vi "BasicHostExampleWithIFw.vi"() -> ()   [LabVIEW 2015]
uses:
  QuadEncInterface/Configuration.ctl
  <vilib>/FPGAPlugInAG/sbRIO-9607/niLvFpga_Open_sbRIO-9607.vi
  <vilib>/rvi/interface/common/dynamic/niFpgaDynamicAddResources.vi
  <vilib>/Utility/error.llb/Error Cluster From Error Code.vi
  <vilib>/rvi/errors/niLvFpgaAdjustHostInterfaceError.vi
  <vilib>/FPGAPlugInAG/Dynamic/niLvFpga_Close_Dynamic.vi
  <vilib>/rvi/interface/nirviOpenFPGA/nirviOpenFPGA.xnode
  Bitfiles/QuadEncdev_FPGATarget_BasicExampleWith_hsZfjqvEqKo.lvbitx
  BasicExampleWithIFw.vi
  <vilib>/rvi/interface/nirviReadWriteControl/nirviReadWriteControl.xnode
  <vilib>/rvi/interface/nirviCloseFPGA/nirviCloseFPGA.xnode
  <instrlib>/_niInstr/FIFO Register Bus/v1/Host/niInstr FIFO Register Bus v1 Host.lvclass
  QuadEncInterface/QuadEncInterface.lvlib
  NiFpgaLv.dll
  <vilib>/rvi/interface/Simulation/niFpgaSimulationCallBeginRW.vi
  <instrlib>/_niInstr/Instruction Framework/v1/Host/Subsystem Map/niInstr Subsystem Map v1 Host.lvclass
panel:
  in  "stop":bool
  out "AbsPosition":i32
  out "RevPosition":i32
  out "CW_direction":bool
  out "Output":T1
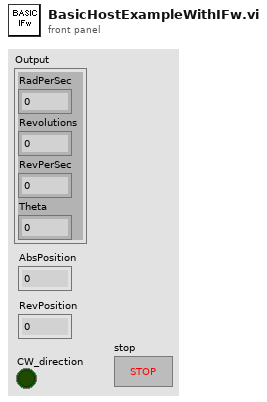
[diagram p1: front panel]
types:
  T1 = cluster{"RadPerSec":sgl, "Revolutions":sgl, "RevPerSec":sgl, "Theta":sgl}
  T2 = typedef "QuadEncInterface.lvlib/Configuration.ctl" = cluster{"ClkRate":dbl, "dT":dbl, "TicksPerRev":u32, "ReversePolarity":bool}
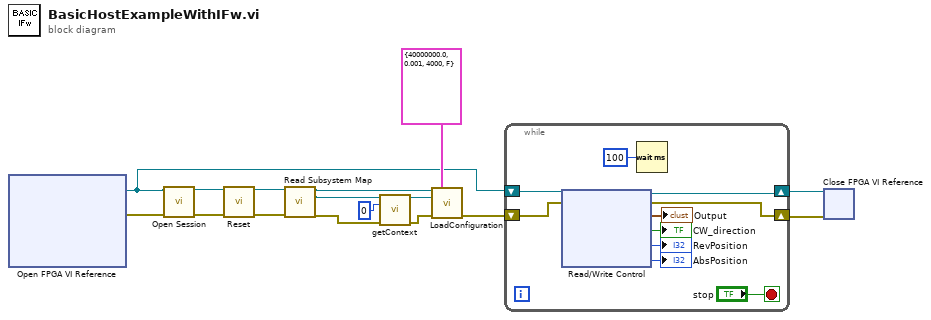
[diagram p0: block diagram]
diagram:
  n1 = xnode "Open FPGA VI Reference"() -> ("FPGA VI Reference Out"=w4:refnum<k20>, "error out"=w5:errorcluster)  [unwired: 2 in]
  n2 = call <instrlib>:"Open Session.vi"("fpga ref"=w4, "error in"=w5) -> ("session out"=w8:refnum<class "niInstr FIFO Register Bus v1 Host.lvclass">, "error out"=w9:errorcluster)  [unwired: 12 in]
  n3 = call-dynamic "Reset.vi"("session in"=w8, "error in"=w9) -> ("session out"=w6:refnum<class "niInstr FIFO Register Bus v1 Host.lvclass">, "error out"=w7:errorcluster)  [unwired: 12 in]
  n4 = call <instrlib>:"Read Subsystem Map.vi"("instruction target in"=w6, "error in"=w7) -> ("instruction target out"=w3:refnum<class "niInstr FIFO Register Bus v1 Host.lvclass">, "subsystem map"=w2:refnum<class "niInstr Subsystem Map v1 Host.lvclass">, "error out"=w1:errorcluster)  [unwired: 11 in]
  n5 = call "getContext.vi"("subsystemMap"=w2, "instance"=u8 0, "error in"=w1) -> ("QuadEncContext"=w14:refnum<class "niInstr Instruction Framework Context v1 Host.lvclass">, "error out"=w15:errorcluster)  [unwired: 11 in]
  n6 = call "LoadConfiguration.vi"("instruction target in"=w3, "Configuration"=T2 {"ClkRate"=40000000.0, "dT"=0.001, "TicksPerRev"=4000, "ReversePolarity"=FALSE}, "QuadEncContext in"=w14, "error in (no error)"=w15) -> ("error out"=w12:errorcluster)  [unwired: 9 in, 2 out]
  n7 = while {
    shift-right: [w19] -> w10
    shift-left: w12 -> [w25]
    shift-right: [w24] -> w11
    shift-left: w4 -> [w26]
    stop <- "stop" stop-if-true
    n8 = xnode "Read/Write Control"("FPGA VI Reference In"=w26, "error in"=w25) -> ("FPGA VI Reference Out"=w24:refnum<k20>, "error out"=w19:errorcluster, "Output"=→"Output":T1, "CW_direction"=→"CW_direction":bool, "RevPosition"=→"RevPosition":i32, "AbsPosition"=→"AbsPosition":i32)
    n9 = Wait (ms)(milliseconds to wait=u32 100) -> ()  [unwired: 1 out]
  }
  n10 = xnode "Close FPGA VI Reference"("FPGA VI Reference In"=w11, "error in"=w10) -> ()  [unwired: 1 out]
